vi "compute rates.vi"(0 "Host Plot Controls":T3={"refresh"=FALSE, "PMTs for Host"={"Sa"=1, "Sb"=0, "g-factor"=1}, "Peaks"={"# bins"=100, "min"=0.0, "max"=10.0}, "Averages"={"# bins"=100, "max"=10.0, "min"=0.0}, "Durations"={"# bins"=100, "max"=10.0, "min"=0.0}, "FP-FPGA"={"# bins"=100, "max"=50.0, "min"=0.0}, "FP-Host"={"# bins"=100, "max"=12.0, "min"=8.0}}, 1 "Time [s]":sgl format="%.1f", 7 "peaks data":T2, 12 "input cluster":T1, 13 "turn off counter":bool) -> (2 "dropfreq":dbl, 3 "sortfreq":dbl, 4 "number detected":i32, 6 "number sorted":dbl, 14 "output cluster":T1)   [LabVIEW 2009]
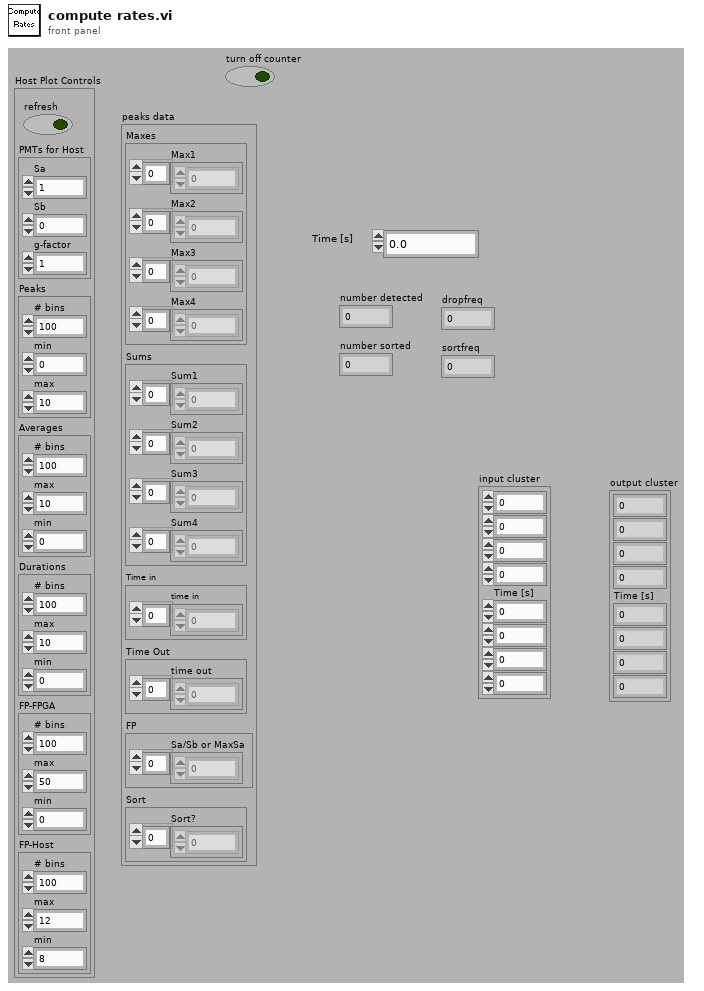
[diagram p1: front panel]
types:
  T1 = cluster{i32, dbl, i32, i32, "Time [s]":sgl, sgl, dbl, dbl}
  T2 = cluster{"Maxes":cluster{"Max1":dbl[], "Max2":dbl[], "Max3":dbl[], "Max4":dbl[]}, "Sums":cluster{"Sum1":dbl[], "Sum2":dbl[], "Sum3":dbl[], "Sum4":dbl[]}, "Time in":cluster{"time in":dbl[]}, "Time Out":cluster{"time out":dbl[]}, "FP":cluster{"Sa/Sb or MaxSa":dbl[]}, "Sort":cluster{"Sort?":dbl[]}}
  T3 = cluster{"refresh":bool, "PMTs for Host":cluster{"Sa":i8, "Sb":i8, "g-factor":i32}, "Peaks":cluster{"# bins":i32, "min":dbl, "max":dbl}, "Averages":cluster{"# bins":i32, "max":dbl, "min":dbl}, "Durations":cluster{"# bins":i32, "max":dbl, "min":dbl}, "FP-FPGA":cluster{"# bins":i32, "max":dbl, "min":dbl}, "FP-Host":cluster{"# bins":i32, "max":dbl, "min":dbl}}
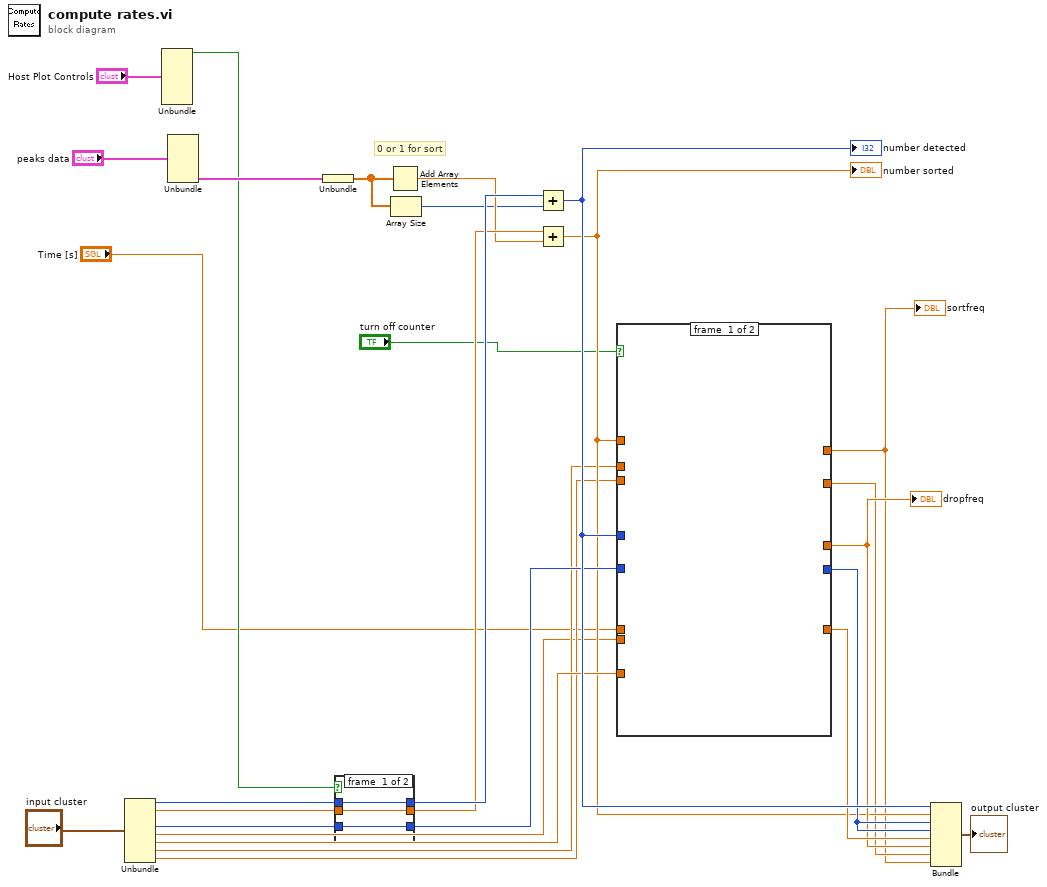
[diagram p0: block diagram]
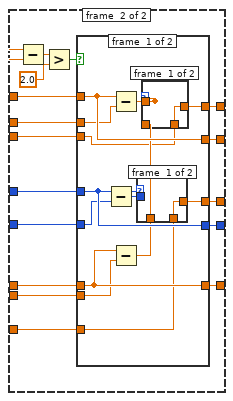
[diagram p2: hidden frame]
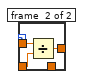
[diagram p3: hidden frame]
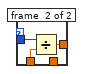
[diagram p4: hidden frame]
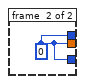
[diagram p6: hidden frame]
diagram:
  # "0 or 1 for sort"
  n1 = Unbundle("input cluster") -> (w17:i32, w18:dbl, w16:i32, "Time [s]"=w2:sgl, w12:sgl, w6:dbl, w5:dbl)  [unwired: 1 out]
  n2 = Unbundle("Host Plot Controls") -> ("refresh"=w20:bool)  [unwired: 6 out]
  n3 = Unbundle("peaks data") -> ("Sort"=w26:cluster{"Sort?":dbl[]})  [unwired: 5 out]
  n4 = Unbundle(w26) -> ("Sort?"=w23:dbl[])
  n5 = case shown="False" w20 {
    tunnel: w17 -> [w31 _]
    tunnel: w18 -> [w30 _]
    tunnel: [w31 w32] -> w25
    tunnel: [w30 w32] -> w24
    tunnel: w16 -> [w29 _]
    tunnel: [w29 w32] -> w15
    frame #0 {
    }
    frame #1 {
      w32 = 0
    }
  }
  n6 = Add Array Elements(numeric array=w23) -> (sum=w22:dbl)
  n7 = Array Size(array=w23) -> (size(s)=w21:i32)
  n8 = Add(x=w25, y=w21) -> (x+y=w19:i32)
  "number detected" <- w19
  n9 = Add(x=w24, y=w22) -> (x+y=w10:dbl)
  "number sorted" <- w10
  n10 = case shown="True" "turn off counter" {
    tunnel: w19 -> [_ w48]
    tunnel: w15 -> [_ w47]
    tunnel: [_ w46] -> w14
    tunnel: [_ w45] -> w13
    tunnel: w12 -> [_ w44]
    tunnel: [_ w43] -> w11
    tunnel: w10 -> [_ w42]
    tunnel: [_ w41] -> w9
    tunnel: w6 -> [_ w40]
    tunnel: w5 -> [_ w39]
    tunnel: [_ w38] -> w4
    tunnel: "Time [s]" -> [_ w37]
    tunnel: w2 -> [_ w36]
    frame #0 {
    }
    frame #1 {
      n11 = Subtract(x=w37, y=w36) -> (x-y=w35:sgl)
      n12 = Greater?(x=w35, y=sgl 2.0 ("x")) -> (0:w34:bool)
      n13 = case shown="True" w34 {
        tunnel: w48 -> [w61 _]
        tunnel: [w61 w74] -> w46
        tunnel: w47 -> [w60 w74]
        tunnel: w37 -> [w59 _]
        tunnel: [w59 w73] -> w45
        tunnel: w36 -> [w58 w73]
        tunnel: [w57 w72] -> w43
        tunnel: w44 -> [w51 w72]
        tunnel: w42 -> [w56 _]
        tunnel: [w56 w70] -> w41
        tunnel: [w54 w71] -> w38
        tunnel: w40 -> [w53 w70]
        tunnel: w39 -> [w49 w71]
        frame #0 {
          n14 = Subtract(x=w61, y=w60) -> (x-y=w52:i32)
          n15 = Subtract(x=w56, y=w53) -> (x-y=w50:dbl)
          n16 = Subtract(x=w59, y=w58) -> (x-y=w55:sgl)
          n17 = case shown="Default" w52 {
            tunnel: w52 -> [_ w69]
            tunnel: [w66 w68] -> w57
            tunnel: w55 -> [_ w67]
            tunnel: w51 -> [w66 _]
            frame #0 {
            }
            frame #1 {
              n18 = Divide(x=w69, y=w67) -> (x/y=w68:sgl)
            }
          }
          n19 = case shown="Default" w50 {
            tunnel: w50 -> [_ w65]
            tunnel: w55 -> [_ w64]
            tunnel: [w62 w63] -> w54
            tunnel: w49 -> [w62 _]
            frame #0 {
            }
            frame #1 {
              n20 = Divide(x=w65, y=w64) -> (x/y=w63:dbl)
            }
          }
        }
        frame #1 {
        }
      }
    }
  }
  "sortfreq" <- w4
  "dropfreq" <- w11
  n21 = Bundle(w19, w10, w14, w14, "Time [s]"=w13, w11, w9, w4) -> (→"output cluster":T1)  [unwired: 1 in]
